vi "Do.vi"(8 "error in (no error)":errorcluster, 10 "Actor in":refnum<class "Actor.lvclass">, 11 "RegisterForMessageSpecificType Msg":refnum<class "RegisterForMessageSpecificType Msg.lvclass">) -> (0 "error out":errorcluster, 2 "Actor out":refnum<class "Actor.lvclass">)   [LabVIEW 2020, in "MailboxManager.lvlib" / "RegisterForMessageSpecificType Msg.lvclass"]
doc: "This VI delivers the message to the actor by calling the appropriate method(s) on the actor."
uses:
  RegisterForMessageSpecificType Msg.lvclass
  <vilib>/ActorFramework/Actor/Actor.lvclass
  RegisterForMessageSpecificType Msg.lvclass/RegisterForMessageSpecificType Msg.ctl
  9ef47adc-f318-494c-9b8b-6df3216d6863.vi
  MailboxManager/MailboxManager.lvclass
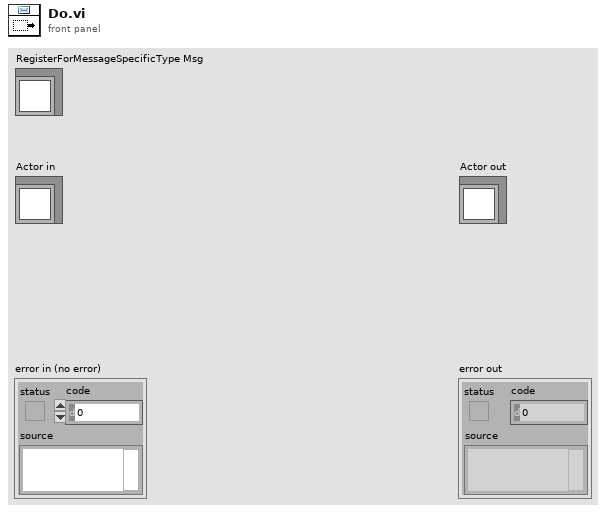
[diagram p1: front panel]
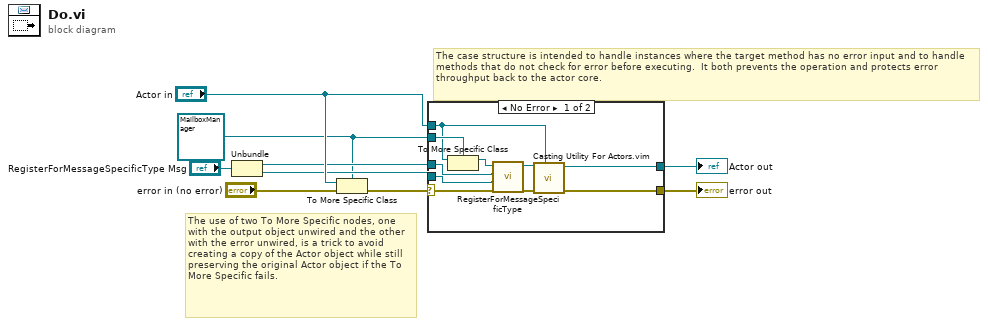
[diagram p0: block diagram]
diagram:
  w1 = refnum<class "MailboxManager.lvclass"> refnum ("MailboxManager.lvlib:MailboxManager.lvclass")
  # "The use of two To More Specific nodes, one with the output object unwired and the other with the error unwired, is a trick to avoid creating a copy of the Actor object while still preserving the original Actor object if the To More Specific fails."
  # "The case structure is intended to handle instances where the target method has no error input and to handle methods that do not check for error before executing.  It both prevents the operation and protects error throughput back to the actor core."
  n1 = Unbundle("RegisterForMessageSpecificType Msg") -> (w3:refnum<class "MailBoxMessage.lvclass">, w2:refnum<class "Message Enqueuer.lvclass">)
  n2 = To More Specific Class(target class=w1, reference="Actor in", error in="error in (no error)") -> (error out=w7:errorcluster)  [unwired: 1 out]
  n3 = case shown="No Error" w7 {
    selector: w7 -> [w15 w21]
    tunnel: [w16 w21] -> w6
    tunnel: [w17 w20] -> w5
    tunnel: "Actor in" -> [w18 w20]
    tunnel: w1 -> [w19 _]
    tunnel: w3 -> [w10 _]
    tunnel: w2 -> [w14 _]
    frame No Error {
      n4 = To More Specific Class(target class=w19, reference=w18) -> (specific class reference=w13:refnum<class "MailboxManager.lvclass">)  [unwired: 1 in, 1 out]
      n5 = call-dynamic "RegisterForMessageSpecificType.vi"("error in (no error)"=w15, "Message Enqueuer"=w14, "Message"=w10, "MailboxManager in"=w13) -> ("error out"=w11:errorcluster, "MailboxManager out"=w12:refnum<class "MailboxManager.lvclass">)  [unwired: 6 in]
      n6 = call "Casting Utility For Actors.vim"("type"=w18, "error in (no error)"=w11, "Actor in"=w12) -> ("error out"=w16:errorcluster, "Actor out"=w17:refnum<class "Actor.lvclass">)  [unwired: 7 in]
    }
    frame Error {
      # "If type check fails, pass the original object out again."
    }
  }
  "error out" <- w6
  "Actor out" <- w5
